vi "Begin.vi"(8 "error in":errorcluster) -> (0 "error out":errorcluster)   [LabVIEW 2016]
doc: "Called before other user functions, this VI is expected to open initial I/O refnums, load in file data, and do all program initialization. Notice that the <B>error out</B> terminal is simply used for data flow. Wiring it to other structures or subVIs ensures that this VI runs first."
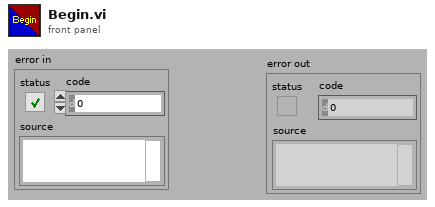
[diagram p1: front panel]
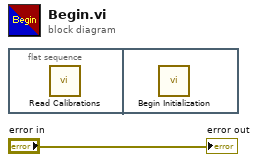
[diagram p0: block diagram]
diagram:
  n1 = flat-sequence {
    frame #0 {
      n2 = call "Read Calibrations.vi"() -> ()  [unwired: 12 in]
    }
    frame #1 {
      n3 = call "Begin Initialization.vi"() -> ()  [unwired: 12 in]
    }
  }
  "error out" <- "error in"
